vi "SCLN_SetShutdownFlagvi.vi"   [LabVIEW 2015]
uses:
  SCLN_RW_Select.ctl
  SCLN_NOTIF_Select.ctl
types:
  T1 = typedef "SCLN_NOTIF_Select.ctl" = enum16{"Server1", "Server2", "Server3", "Server4", "Server5", "Server6", "Server7", "Client1", "Client2", "Client3", "Client4", "Client5", "Client6", "Client7", "Client8", "Client9", "Client10", "Shutdown", "Init_Ready"}
  T2 = typedef "SCLN_RW_Select.ctl" = enum16{"Read", "Write"}
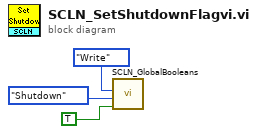
[diagram p0: block diagram]
diagram:
  n1 = call "SCLN_GlobalBooleans.vi"("Write Value"=TRUE, "Element"=SCLN_NOTIF_Select."Shutdown" ("Dome String Ctrl"), "Operation"=SCLN_RW_Select."Write" ("GBL_RW")) -> ()  [unwired: 1 in, 2 out]
